vi "Close.vi"(0 "RS NRPx Power Meter in":refnum<class "Power Meter.lvclass">, 11 "error in":errorcluster) -> (4 "RS NRPx Power Meter out":refnum<class "Power Meter.lvclass">, 15 "error out":errorcluster)   [LabVIEW 2023, in "RS NRPx Power Meter.lvlib" / "Power Meter.lvclass"]
uses:
  Power Meter.lvclass
  Power Meter.lvclass/Power Meter.ctl
  <instrlib>/Rohde&Schwarz Power Meter/Rohde&Schwarz Power Meter.lvlib
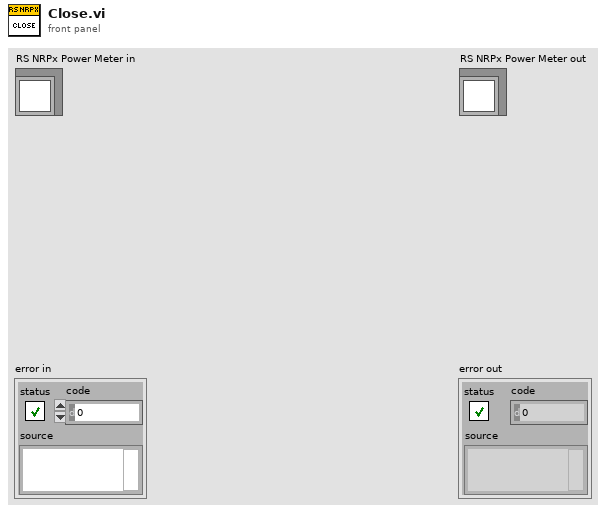
[diagram p1: front panel]
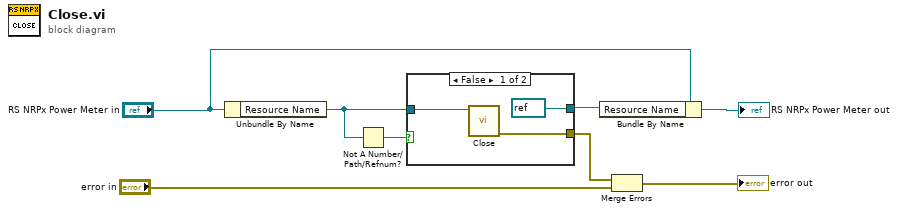
[diagram p0: block diagram]
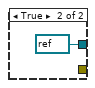
[diagram p2: hidden frame]
diagram:
  n1 = Unbundle By Name("RS NRPx Power Meter in") -> ("Resource Name"=w2:refnum<visa-resource-name>)
  n2 = Not A Number/Path/Refnum?(number/path/refnum=w2) -> (NaN/Path/Refnum?=w4:bool)
  n3 = case shown="False" w4 {
    tunnel: w2 -> [w11 _]
    tunnel: [w10 _] -> w3
    tunnel: [refnum<visa-resource-name> refnum ("Resource Name") refnum<visa-resource-name> refnum ("Resource Name")] -> w1
    frame False {
      n4 = call <instrlib>:"Close.vi"("VISA resource name"=w11) -> ("error out"=w10:errorcluster)  [unwired: 10 in]
    }
    frame True {
    }
  }
  n5 = Bundle By Name(cluster="RS NRPx Power Meter in", "Resource Name"=w1) -> (→"RS NRPx Power Meter out":refnum<class "Power Meter.lvclass">)
  n6 = Merge Errors(w3, "error in") -> (→"error out":errorcluster)
